vi "Simple State Machine template.vi"() -> ()   [LabVIEW 2020]
panel:
  in  "Exit":bool
  in  "Save ConfigFile":bool
  in  "Load ConfigFile":bool
  out "error out":errorcluster
  in  "error in (no error)":errorcluster
  # "XML Configuration File"
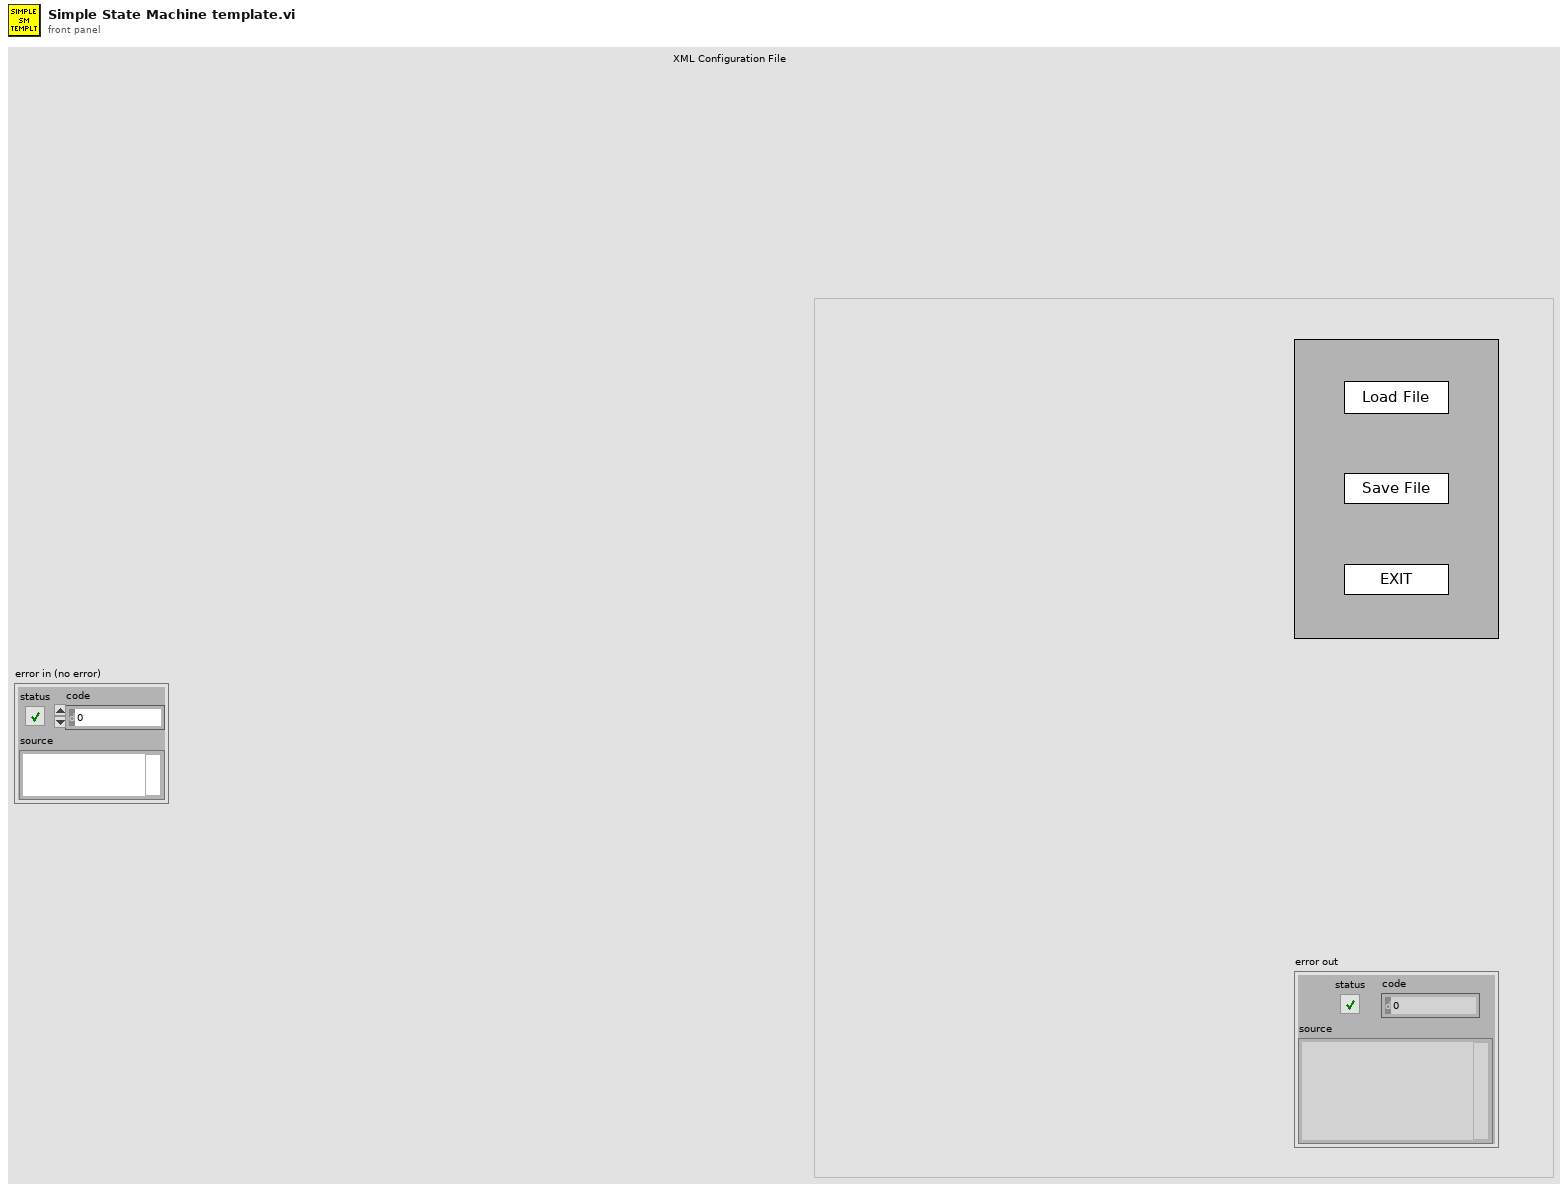
[diagram p1: front panel]
types:
  T1 = enum32{"Invalid", "Standard", "Closed", "Hidden", "Minimized", "Maximized"}
  T2 = cluster{"Core":cluster{"Current VI Reference":refnum<vi>, "Close Panel on Exit?":bool}, "WyPtDictNode":cluster{"Idx":i32, "Cmd Number":string, "Waypoint List":string, "Description":string}[]}
  T3 = cluster{"Idx":i32, "Cmd Number":string, "Waypoint List":string, "Description":string}[]
  T4 = cluster{"Current VI Reference":refnum<vi>, "Close Panel on Exit?":bool}
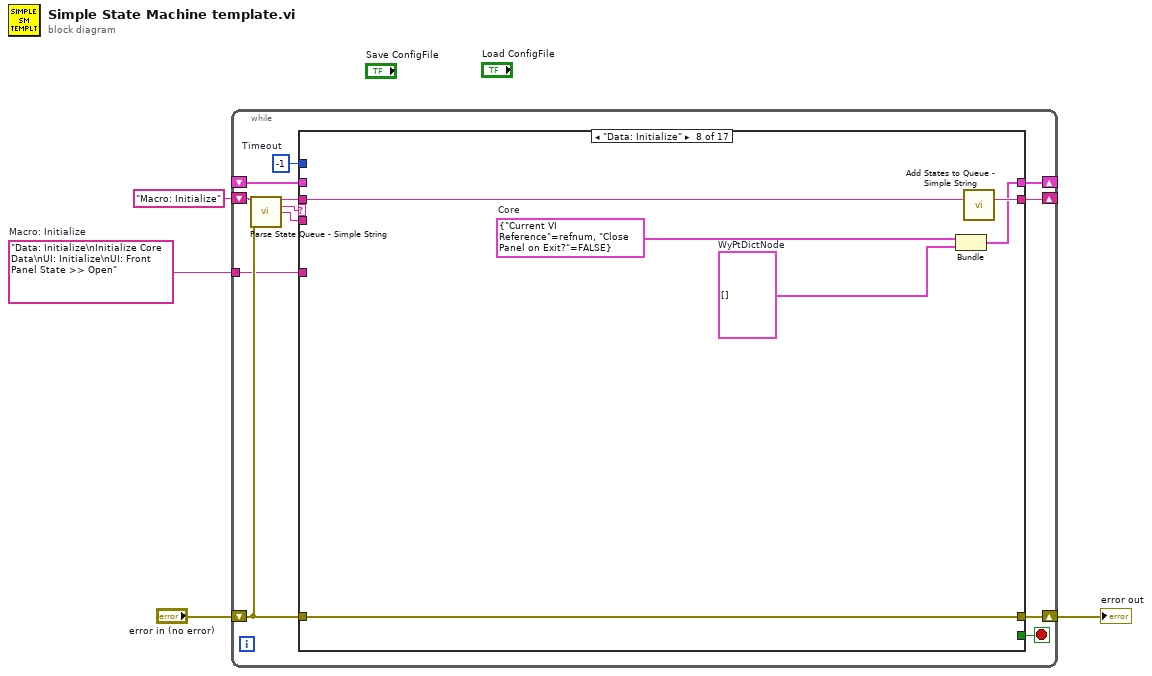
[diagram p0: block diagram]
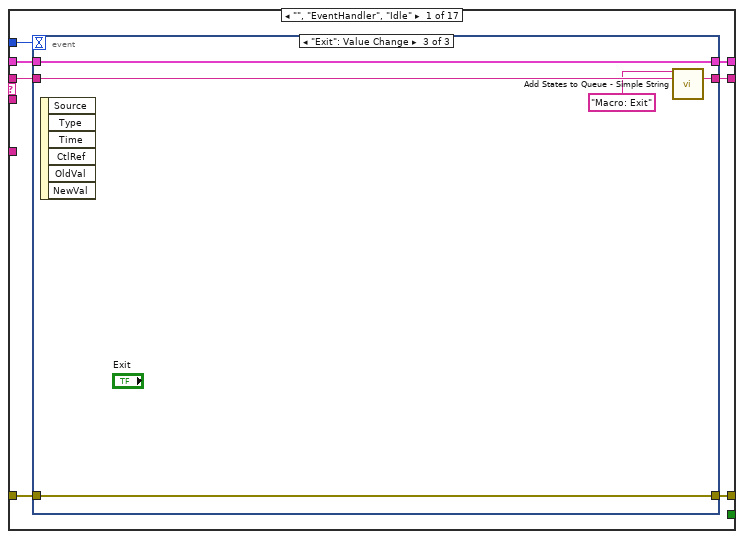
[diagram p2: hidden frame]
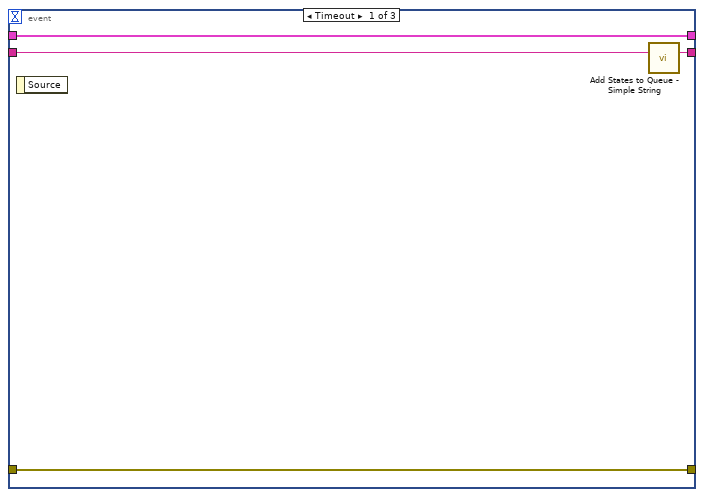
[diagram p3: hidden frame]
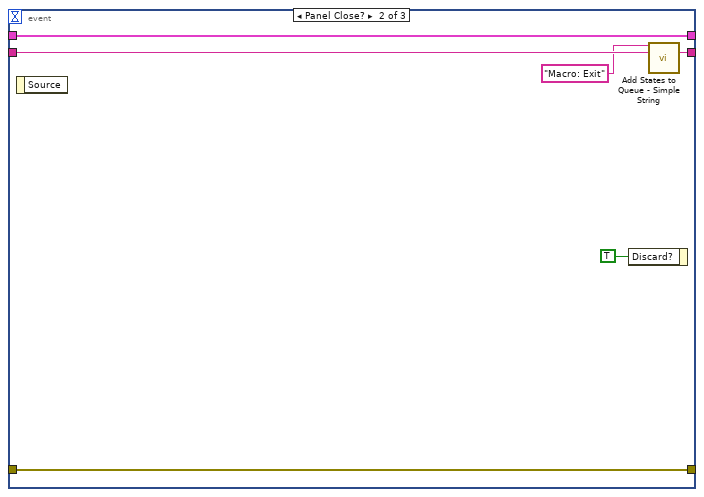
[diagram p4: hidden frame]
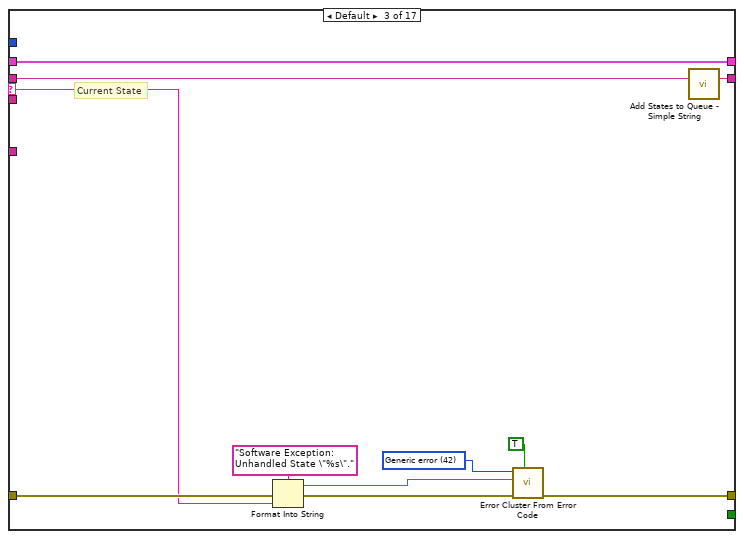
[diagram p6: hidden frame]
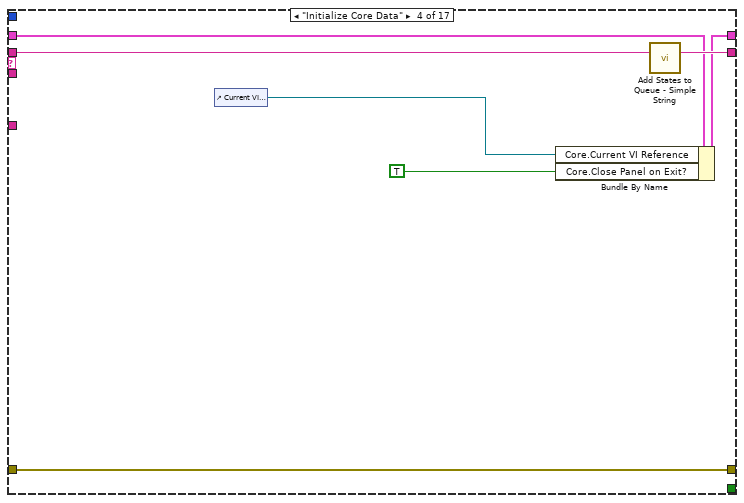
[diagram p7: hidden frame]
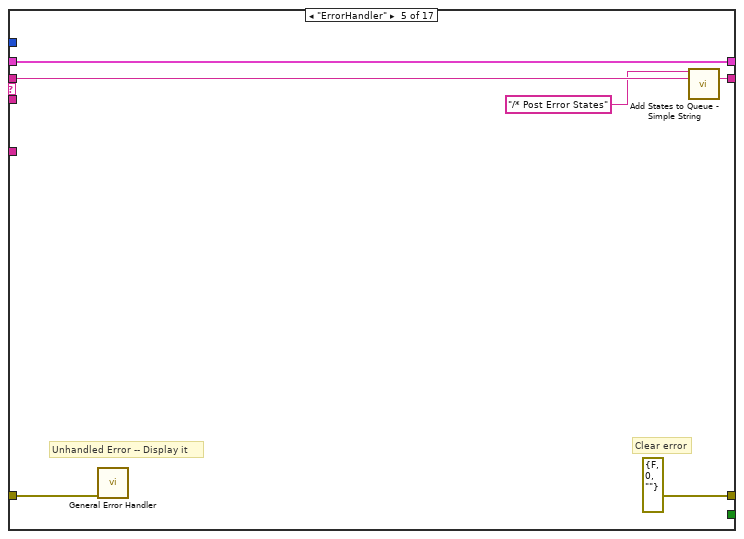
[diagram p8: hidden frame]
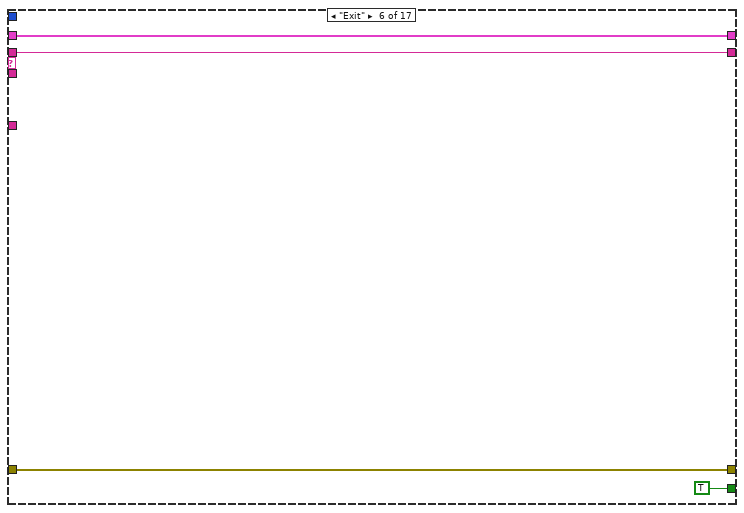
[diagram p9: hidden frame]
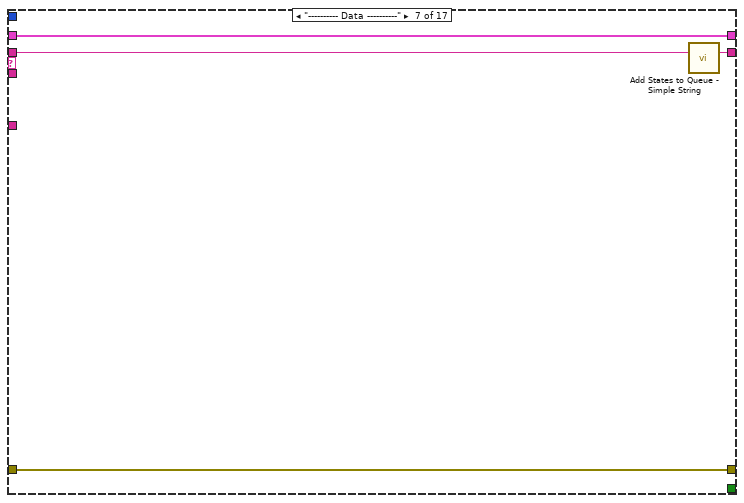
[diagram p10: hidden frame]
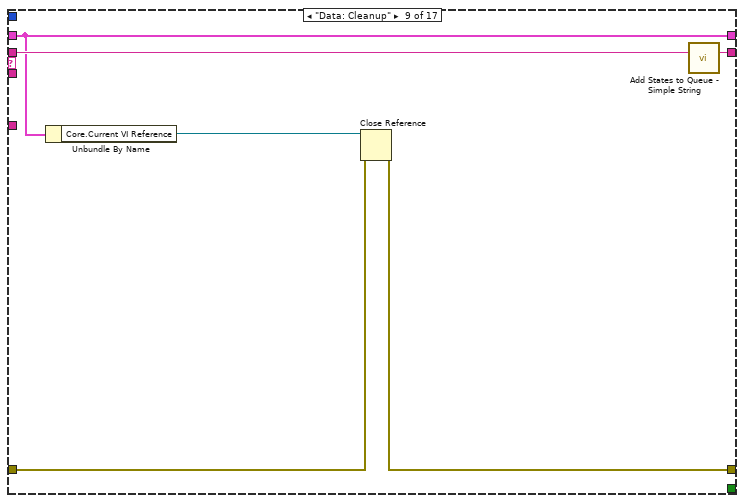
[diagram p11: hidden frame]
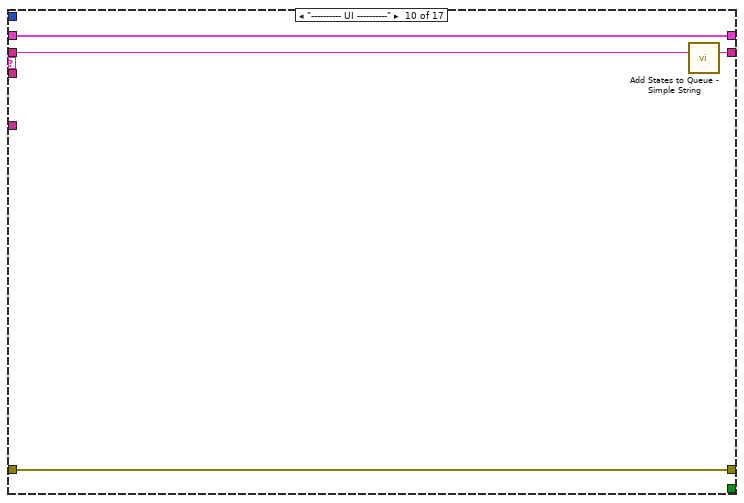
[diagram p12: hidden frame]
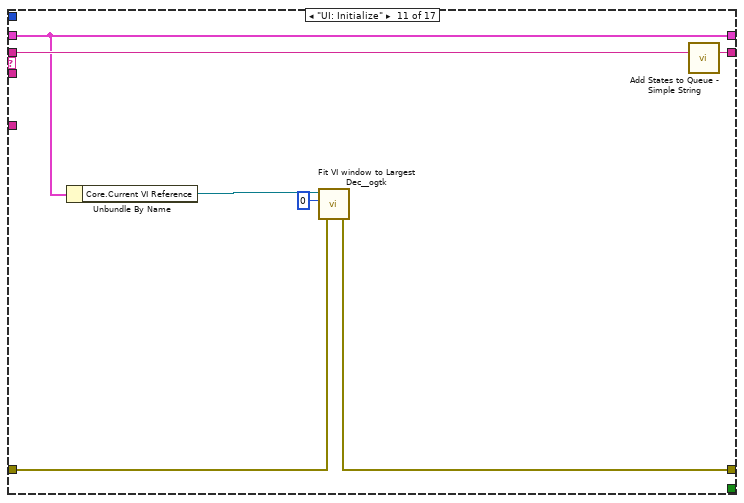
[diagram p13: hidden frame]
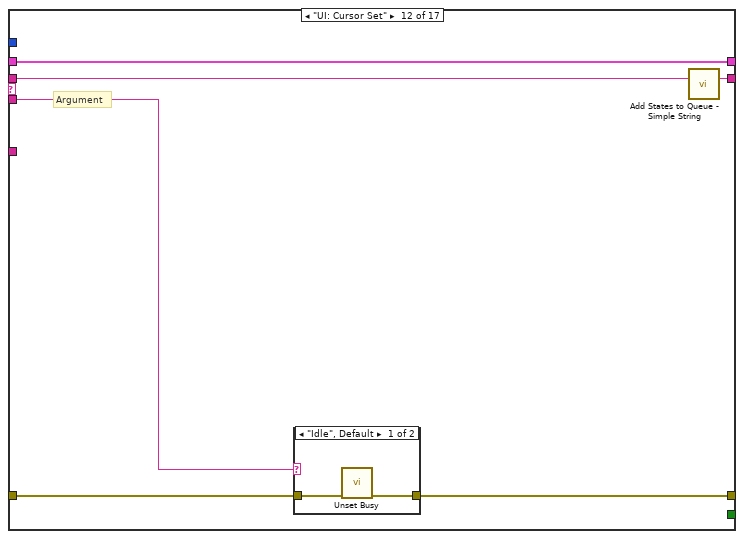
[diagram p14: hidden frame]
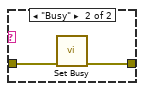
[diagram p15: hidden frame]
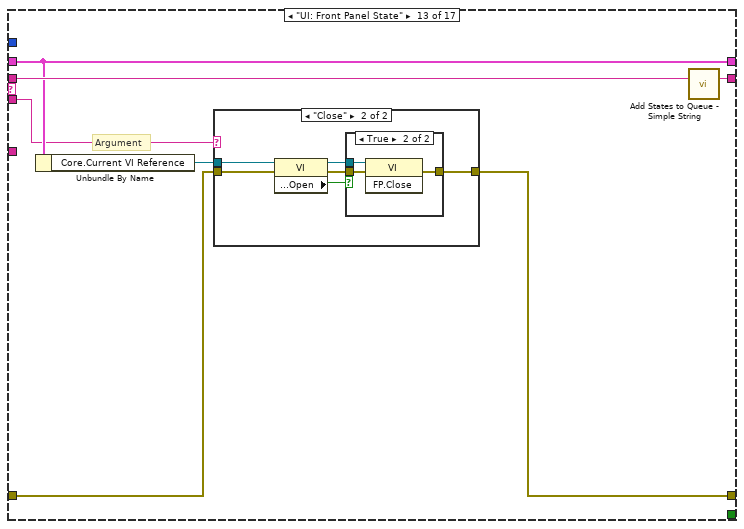
[diagram p16: hidden frame]
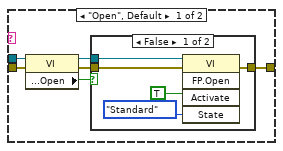
[diagram p17: hidden frame]
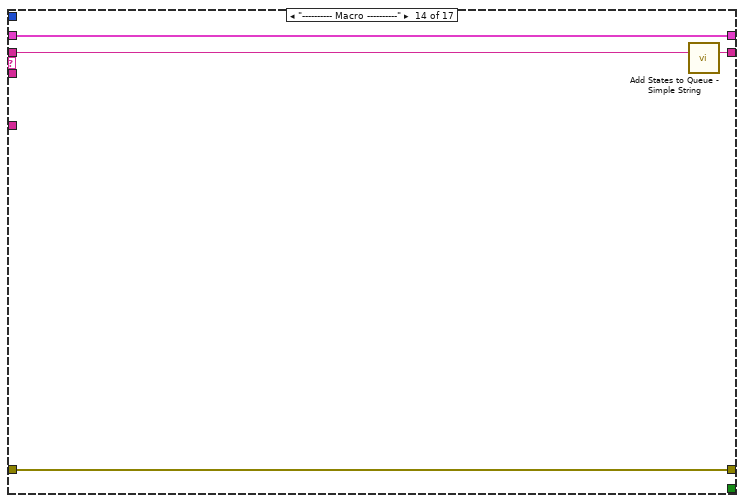
[diagram p20: hidden frame]
diagram:
  w1 = "Data: Initialize\nInitialize Core Data\nUI: Initialize\nUI: Front Panel State >> Open"  # Macro: Initialize
  n1 = while {
    shift-right: [w9] -> _
    shift-left: _ -> [w8]
    shift-right: [w12] -> w3
    shift-left: "error in (no error)" -> [w6]
    shift-right: [w11] -> _
    shift-left: "Macro: Initialize" -> [w13]
    tunnel: w1 -> [w5]
    stop <- w10 stop-if-true
    w7 = -1  # Timeout
    n2 = call <vilib>:"Parse State Queue - Simple String.vi"("StateQ in"=w13, "error"=w6) -> ("Remaining States"=w15:string, "Next State"=w16:string, "Command (Optional)"=w14:string)  [unwired: 9 in, 2 out]
    n3 = case shown="\"Data: Initialize\"" w16 {
      selector: w16 -> [_ _ w42 _ _ _ _ _ _ _ _ _ _ _ _ _ _]
      tunnel: w15 -> [w23 w39 w46 w59 w65 w66 w73 w79 w85 w89 w96 w102 w113 w139 w144 w154 w158]
      tunnel: w14 -> [_ _ _ _ _ _ _ _ _ _ _ w97 w107 _ _ _ _]
      tunnel: w8 -> [w21 w40 w44 w55 w62 w69 w70 _ w80 w86 w94 w100 w109 w136 w141 w151 w155]
      tunnel: [w20 w41 w48 w56 errorcluster {"status"=FALSE, "code"=0, "source"=""} ("error out") w68 w71 w75 w81 w87 w91 w98 w110 w137 w142 w152 w156] -> w12
      tunnel: w6 -> [w19 w41 w47 w56 w61 w68 w71 w75 w82 w87 w90 w99 w111 w137 w142 w152 w156]
      tunnel: [w22 w39 w45 w58 w64 w66 w72 w78 w84 w88 w95 w101 w112 w138 w143 w153 w157] -> w11
      tunnel: [_ _ _ _ _ TRUE _ _ _ _ _ _ _ _ _ _ _] -> w10
      tunnel: [w18 w40 w44 w57 w62 w69 w70 w77 w80 w86 w94 w100 w109 w136 w141 w151 w155] -> w9
      tunnel: w7 -> [w17 _ _ _ _ _ _ _ _ _ _ _ _ _ _ _ _]
      tunnel: w5 -> [_ _ _ _ _ _ _ _ _ _ _ _ _ _ w140 _ _]
      frame "", "EventHandler", "Idle" {
        n4 = event shown="[2] \"Exit\": Value Change" {
          selector: _ -> [_ _ _]
          dyn-events: _ -> [_ _ _]
          timeout: w17 -> [_ _ _]
          tunnel: w23 -> [w27 w33 w38]
          tunnel: [w26 w32 w37] -> w22
          tunnel: w21 -> [w24 w30 w35]
          tunnel: [w25 w31 w36] -> w20
          tunnel: w19 -> [w25 w31 w36]
          tunnel: [w24 w30 w35] -> w18
          event Timeout {
            n5 = event-data() -> ()  [unwired: 1 in, 1 out]
            n6 = call <vilib>:"Add States to Queue - Simple String.vi"("States in"=w27) -> ("States out"=w26:string)  [unwired: 14 in]
          }
          event Panel Close? {
            n7 = event-data() -> ()  [unwired: 1 in, 1 out]
            n8 = event-data("Discard?"=TRUE) -> ()  [unwired: 1 in, 1 out]
            n9 = call <vilib>:"Add States to Queue - Simple String.vi"("States in Front"="Macro: Exit", "States in"=w33) -> ("States out"=w32:string)  [unwired: 13 in]
          }
          event "Exit": Value Change {
            n10 = event-data() -> ()  [unwired: 1 in, 6 out]
            n11 = call <vilib>:"Add States to Queue - Simple String.vi"("States in Front"="Macro: Exit", "States in"=w38) -> ("States out"=w37:string)  [unwired: 13 in]
          }
        }
      }
      frame "---------- Core ----------" {
      }
      frame Default {
        w51 = 42 items=["No error", "Argument error", "Memory is full", "Out of zone", "End of file", "File already open", "Generic file I/O error", "File not found", "File permission error", "Disk is full", "Duplicate path", "Too many files open", "System feature not enabled", "Resource file not found", "Cannot add resource", "Resource not found", "Image not found", "Image memory error", "Pen does not exist", "Config type invalid", "Config token not found", "Config parse error", "Config memory error", "Bad external code format", "Bad external code offset", "External code not present", "Null window", "Destroy window error", "Null menu", "Print aborted", "Bad print record", "Print driver error", "Windows error during printing", "Memory error during printing", "Print dialog error", "Generic print error", "Invalid device refnum", "Device not found", "Device parameter error", "Device unit error", "Cannot open device", "Device call aborted", "Generic error", "Cancelled by user", "Object ID too low", "Object ID too high", "Object not in heap", "Unknown heap", "Unknown object (invalid DefProc)", "Unknown object (DefProc not in table)", "Message out of range", "Invalid (null) method", "Unknown message", "Manager call not supported", "Bad address", "Network operation in progress", "Network operation timed out", "Connection is busy", "Network attribute not supported", "Network error", "Address in use", "System out of memory", "Connection aborted", "Connection refused", "Not connected", "Already connected", "Connection closed", "Initialization error (interapplication manager)", "Bad occurrence", "Wait on unbound occurrence handler", "Occurrence queue overflow", "Datalog type conflict", "Unused", "Unrecognized type (interapplication manager)", "Memory corrupt", "Failed to make temporary DLL", "Old CIN version", "Drag socket not found", "Failed to load drop-object", "Failed to register OLE object", "Failed to release OLE object", "Format specifier type mismatch", "Unknown format specifier", "Too few format specifiers", "Too many format specifiers", "Scan failed", "Newer CIN version", "Error converting to variant", "Runtime menu error", "Password tampered", "Variant attribute not found", "Incompatible variant data type", "Event data is not available", "Event Store is not present", "Occurrence is not found", "Event Queue is not created", "Event info is not available", "Refnum passed is NULL", "Error retrieving Class GUID", "Error retrieving CoClass GUID", "Error retrieving TypeLib GUID.", "Bad built application magic bytes.", "Specific driver is different from the specific driver associated with the Logical Name.", "There is no session opened to the class driver.", "Max Error", "MAX - Error with config objects", "MAX - Error loading configuration", "MAX - Group not supported"]
        # "Current State"
        n12 = Format Into String(format string="Software Exception: Unhandled State \"%s\"." ("message"), error in=w47, w42) -> (resulting string=w50:string, error out=w49:errorcluster)  [unwired: 1 in]
        n13 = call <vilib>:"Error Cluster From Error Code.vi"("show call chain? (False)"=TRUE, "error in (no error)"=w49, "error message (\"\")"=w50, "error code (0)"=w51) -> ("error out"=w48:errorcluster)  [unwired: 5 in]
        n14 = call <vilib>:"Add States to Queue - Simple String.vi"("States in"=w46) -> ("States out"=w45:string)  [unwired: 14 in]
      }
      frame "Initialize Core Data" {
        n15 = control-ref of="Current VI Reference"() -> (w54:refnum<vi>)
        n16 = Bundle By Name(cluster=w55, "Core.Current VI Reference"=w54, "Core.Close Panel on Exit?"=TRUE) -> (w57:T2)
        n17 = call <vilib>:"Add States to Queue - Simple String.vi"("States in"=w59) -> ("States out"=w58:string)  [unwired: 14 in]
      }
      frame "ErrorHandler" {
        # "Unhandled Error -- Display it"
        # "Clear error"
        n18 = call <vilib>:"General Error Handler.vi"("error in (no error)"=w61) -> ()  [unwired: 10 in, 5 out]
        n19 = call <vilib>:"Add States to Queue - Simple String.vi"("States in Front"="/* Post Error States", "States in"=w65) -> ("States out"=w64:string)  [unwired: 13 in]
      }
      frame "Exit" {
      }
      frame "---------- Data ----------" {
        n20 = call <vilib>:"Add States to Queue - Simple String.vi"("States in"=w73) -> ("States out"=w72:string)  [unwired: 14 in]
      }
      frame "Data: Initialize" {
        w74 = T3 []  # WyPtDictNode
        w76 = T4 {"Current VI Reference"=refnum, "Close Panel on Exit?"=FALSE}  # Core
        n21 = Bundle("Core"=w76, "WyPtDictNode"=w74) -> (w77:T2)  [unwired: 1 in]
        n22 = call <vilib>:"Add States to Queue - Simple String.vi"("States in"=w79) -> ("States out"=w78:string)  [unwired: 14 in]
      }
      frame "Data: Cleanup" {
        n23 = Unbundle By Name(w80) -> ("Core.Current VI Reference"=w83:refnum<vi>)
        n24 = Close Reference(reference=w83, error in (no error)=w82) -> (error out=w81:errorcluster)
        n25 = call <vilib>:"Add States to Queue - Simple String.vi"("States in"=w85) -> ("States out"=w84:string)  [unwired: 14 in]
      }
      frame "---------- UI ----------" {
        n26 = call <vilib>:"Add States to Queue - Simple String.vi"("States in"=w89) -> ("States out"=w88:string)  [unwired: 14 in]
      }
      frame "UI: Initialize" {
        n27 = Unbundle By Name(w94) -> ("Core.Current VI Reference"=w93:refnum<vi>)
        n28 = call <userlib>:"Fit VI window to Largest Dec__ogtk.vi"("error in (no error)"=w90, "border spacing (2 px)"=0, "VI Ref (calling VI)"=w93) -> ("error out"=w91:errorcluster)  [unwired: 3 in, 1 out]
        n29 = call <vilib>:"Add States to Queue - Simple String.vi"("States in"=w96) -> ("States out"=w95:string)  [unwired: 14 in]
      }
      frame "UI: Cursor Set" {
        # "Argument"
        n30 = case shown="\"Idle\", Default" w97 {
          tunnel: w99 -> [w104 w106]
          tunnel: [w103 w105] -> w98
          frame "Idle", Default {
            n31 = call <vilib>:"Unset Busy.vi"("error in (no error)"=w104) -> ("error out"=w103:errorcluster)  [unwired: 10 in]
          }
          frame "Busy" {
            n32 = call <vilib>:"Set Busy.vi"("error in (no error)"=w106) -> ("error out"=w105:errorcluster)  [unwired: 9 in, 1 out]
          }
        }
        n33 = call <vilib>:"Add States to Queue - Simple String.vi"("States in"=w102) -> ("States out"=w101:string)  [unwired: 14 in]
      }
      frame "UI: Front Panel State" {
        # "Argument"
        n34 = Unbundle By Name(w109) -> ("Core.Current VI Reference"=w108:refnum<vi>)
        n35 = case shown="\"Close\"" w107 {
          tunnel: w111 -> [w117 w130]
          tunnel: [w119 w131] -> w110
          tunnel: w108 -> [w118 w128]
          frame "Open", Default {
            n36 = property class="VI"(reference=w118, error in=w117) -> (reference out=w115:refnum<vi>, error out=w116:errorcluster, "Front Panel.Open"=w114:bool)
            n37 = case shown="False" w114 {
              tunnel: [w122 w125] -> w119
              tunnel: w116 -> [w121 w125]
              tunnel: w115 -> [w120 _]
              frame False {
                n38 = invoke class="VI" method="FP.Open"(reference=w120, error in=w121, "Activate"=TRUE, "State"=T1."Standard") -> (error out=w122:errorcluster)  [unwired: 1 in, 4 out]
              }
              frame True {
              }
            }
          }
          frame "Close" {
            n39 = property class="VI"(reference=w128, error in=w130) -> (reference out=w127:refnum<vi>, error out=w129:errorcluster, "Front Panel.Open"=w126:bool)
            n40 = case shown="True" w126 {
              tunnel: [w132 w135] -> w131
              tunnel: w129 -> [w132 w134]
              tunnel: w127 -> [_ w133]
              frame False {
              }
              frame True {
                n41 = invoke class="VI" method="FP.Close"(reference=w133, error in=w134) -> (error out=w135:errorcluster)  [unwired: 1 in, 2 out]
              }
            }
          }
        }
        n42 = call <vilib>:"Add States to Queue - Simple String.vi"("States in"=w113) -> ("States out"=w112:string)  [unwired: 14 in]
      }
      frame "---------- Macro ----------" {
        n43 = call <vilib>:"Add States to Queue - Simple String.vi"("States in"=w139) -> ("States out"=w138:string)  [unwired: 14 in]
      }
      frame "Macro: Initialize" {
        n44 = call <vilib>:"Add States to Queue - Simple String.vi"("States in Front"=w140, "States in"=w144) -> ("States out"=w143:string)  [unwired: 13 in]
      }
      frame "Macro: Exit" {
        n45 = Unbundle By Name(w151) -> ("Core.Close Panel on Exit?"=w150:bool)
        n46 = Select(t="UI: Front Panel State >> Close", s=w150, f="") -> (s? t:f=w147:string)
        n47 = call <vilib>:"Add States to Queue - Simple String.vi"("States in"=w147, "States at Back"="Data: Cleanup\nExit") -> ("States out"=w145:string)  [unwired: 13 in]
        n48 = call <vilib>:"Add States to Queue - Simple String.vi"("States in Front"=w145, "States in"=w154) -> ("States out"=w153:string)  [unwired: 13 in]
      }
      frame "---------- Action ----------" {
        n49 = call <vilib>:"Add States to Queue - Simple String.vi"("States in"=w158) -> ("States out"=w157:string)  [unwired: 14 in]
      }
    }
  }
  "error out" <- w3
